vi "Project From Point.vi"(9 "distance":dbl, 10 "th":dbl=nan, 11 "Point In":cluster{"x":dbl, "y":dbl, "th":dbl}) -> (3 "Point Out":cluster{"x":dbl, "y":dbl, "th":dbl})   [LabVIEW 2018]
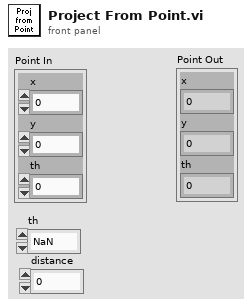
[diagram p1: front panel]
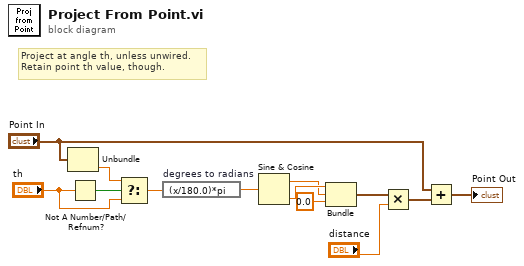
[diagram p0: block diagram]
diagram:
  # "Project at angle th, unless unwired.\nRetain point th value, though."
  n1 = Unbundle("Point In") -> ("th"=w2:dbl)  [unwired: 2 out]
  n2 = Not A Number/Path/Refnum?(number/path/refnum="th") -> (NaN/Path/Refnum?=w5:bool)
  n3 = Select(t=w2, s=w5, f="th") -> (s? t:f=w1:dbl)
  n4 = expression code="(x/180.0)*pi" "degrees to radians"(w1) -> (w10:dbl)
  n5 = Sine & Cosine(0:w10) -> (1:w11:dbl, 2:w12:dbl)
  n6 = Bundle(w12, w11, 0.0) -> (w9:cluster{dbl, dbl, dbl})  [unwired: 1 in]
  n7 = Multiply(x=w9, y="distance") -> (x*y=w7:cluster{dbl, dbl, dbl})
  n8 = Add(x="Point In", y=w7) -> (x+y=→"Point Out":cluster{dbl, dbl, dbl})
